vi "DistanceToTime_mm_us.vi"(9 "Length":dbl, 10 "Start":dbl, 11 "Value":dbl) -> (2 "Numeric":dbl, 3 "Numeric 2":dbl)   [LabVIEW 2026]
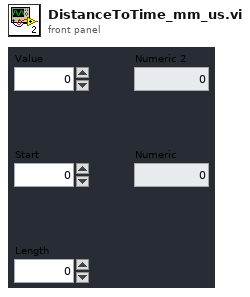
[diagram p1: front panel]
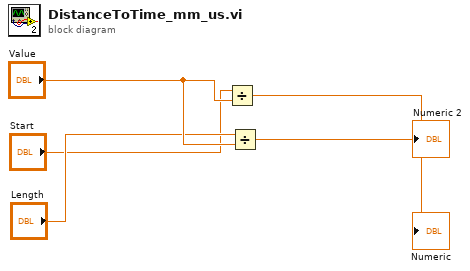
[diagram p0: block diagram]
diagram:
  n1 = Divide(x="Start", y="Value") -> (x/y=→"Numeric":dbl)
  n2 = Divide(x="Length", y="Value") -> (x/y=→"Numeric 2":dbl)
